vi "Error Code Processor.vi"() -> ()   [LabVIEW 2012]
uses:
  <vilib>/Utility/file.llb/Read From Spreadsheet File (string).vi
panel:
  in  "Typedef für Error Labels":path
  in  "Typedef für Error Codes":path
  in  "Btn_ReadErrorFromCsv":bool
  in  "ErrorTable":string[][](table) caption="Codetabelle"
  in  "Btn_SaveErrorToCtl":bool
  in  "Exit":bool
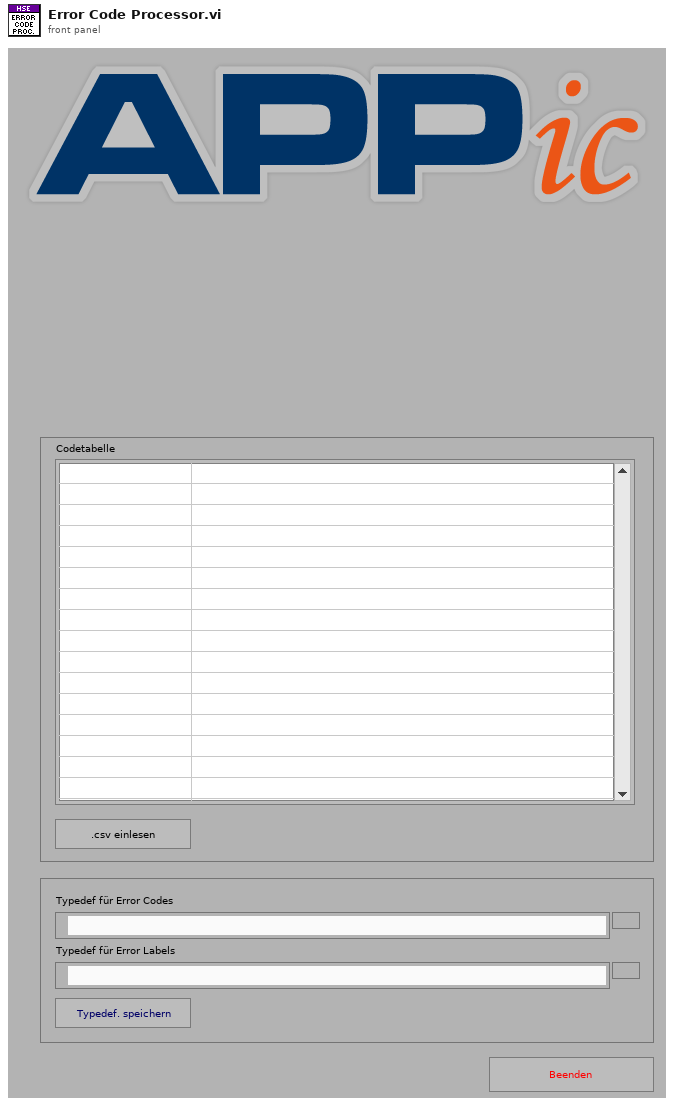
[diagram p1: front panel]
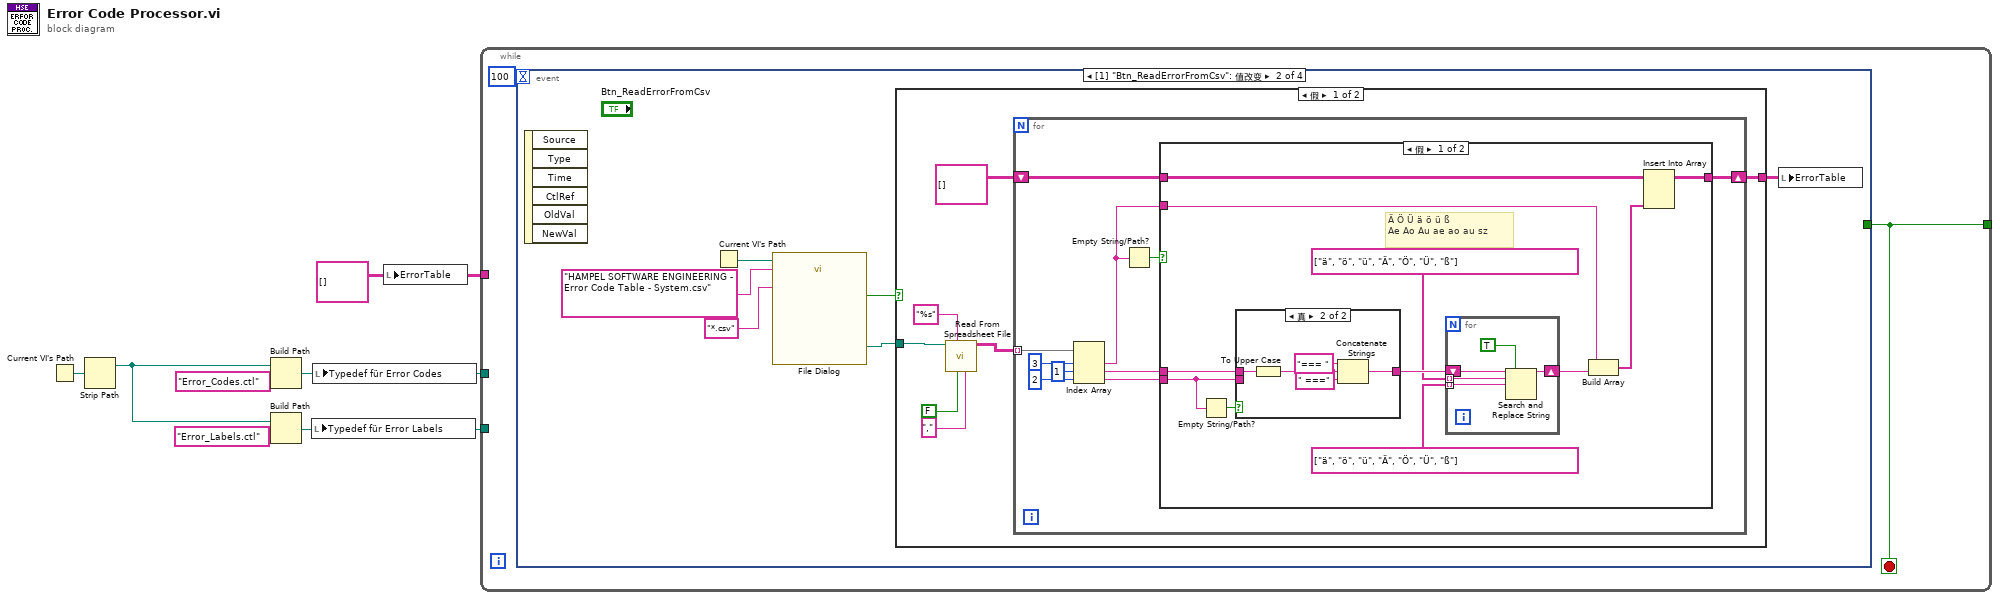
[diagram p0: block diagram]
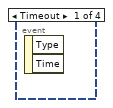
[diagram p2: hidden frame]
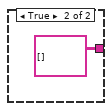
[diagram p5: hidden frame]
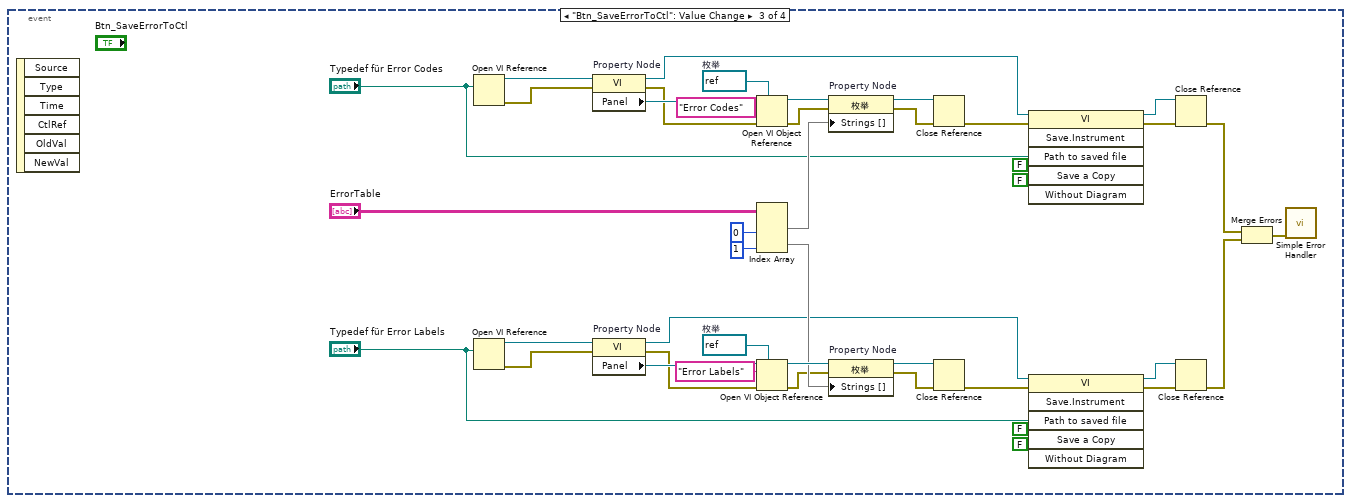
[diagram p6: hidden frame]
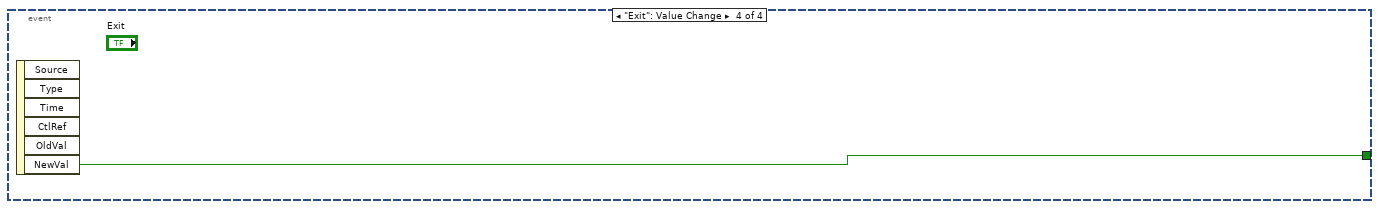
[diagram p7: hidden frame]
diagram:
  w7 = string[][] [] ("ErrorTable")
  n1 = Current VI's Path() -> (path=w6:path)
  n2 = Strip Path(path=w6) -> (stripped path=w1:path)  [unwired: 1 out]
  n3 = Build Path(base path=w1, name or relative path="Error_Codes.ctl") -> (appended path=w5:path)
  n4 = Build Path(base path=w1, name or relative path="Error_Labels.ctl") -> (appended path=w4:path)
  n5 = local write "Typedef für Error Labels"(w4) -> ()
  n6 = local write "Typedef für Error Codes"(w5) -> ()
  n7 = local write "ErrorTable"(w7) -> ()
  n8 = while {
    tunnel: [w9] -> _
    tunnel: w7 -> [_]
    tunnel: w5 -> [_]
    tunnel: w4 -> [_]
    stop <- w9 stop-if-true
    n9 = event shown="[1] \"Btn_ReadErrorFromCsv\": 值改变" {
      selector: _ -> [_ _ _ _]
      dyn-events: _ -> [_ _ _ _]
      timeout: 100 -> [_ _ _ _]
      tunnel: [_ _ _ w99] -> w9
      event Timeout {
        n10 = event-data() -> ()  [unwired: 3 out]
      }
      event "Btn_ReadErrorFromCsv": Value Change {
        n11 = event-data() -> ()  [unwired: 7 out]
        n12 = Current VI's Path() -> (path=w12:path)
        n13 = call "File Dialog"("start path"=w12, "default name"="HAMPEL SOFTWARE ENGINEERING - Error Code Table - System.csv", "pattern (all files)"="*.csv") -> ("selected path"=w14:path, "cancelled"=w13:bool)  [unwired: 9 in, 2 out]
        n14 = case shown="假" w13 {
          tunnel: [w17 string[][] []] -> w15
          tunnel: w14 -> [w16 _]
          frame False {
            n15 = call-poly <vilib>:"Read From Spreadsheet File.vi"("delimiter (\\t)"="," ("delimiter (\\t)"), "transpose (no:F)"=FALSE, "format (%s)"="%s", "file path (dialog if empty)"=w16) -> ("all rows"=w19:string[][])  [unwired: 3 in, 4 out]
            n16 = for {
              tunnel: w19 -> [w32] mode=indexing
              shift-right: [w27] -> w17
              shift-left: string[][] [] -> [w29]
              n17 = Index Array(array=w32, index #1=3 ("index"), index #2=1 ("index"), index #3=2 ("index")) -> (element #1=w25:string, element #2=w24:string, element #3=w23:string)
              n18 = Empty String/Path?(string/path=w25) -> (empty?=w28:bool)
              n19 = case shown="假" w28 {
                tunnel: w29 -> [w43 w55]
                tunnel: w25 -> [w37 _]
                tunnel: [w42 w55] -> w27
                tunnel: w24 -> [w38 _]
                tunnel: w23 -> [w39 _]
                frame False {
                  # "Ä Ö Ü ä ö ü ß\nAe Ao Au ae ao au sz"
                  n20 = Empty String/Path?(string/path=w39) -> (empty?=w40:bool)
                  n21 = case shown="真" w40 {
                    tunnel: w39 -> [w49 _]
                    tunnel: [w49 w53] -> w36
                    tunnel: w38 -> [_ w54]
                    frame False {
                    }
                    frame True {
                      n22 = To Upper Case(1:w54) -> (0:w50:string)
                      n23 = Concatenate Strings("=== " ("string"), w50, " ===" ("string")) -> (w53:string)
                    }
                  }
                  n24 = for {
                    tunnel: string[] ["ä", "ö", "ü", "Ä", "Ö", "Ü", "ß"] -> [w46] mode=indexing
                    shift-right: [w47] -> w35
                    shift-left: w36 -> [w48]
                    tunnel: string[] ["ä", "ö", "ü", "Ä", "Ö", "Ü", "ß"] -> [w45] mode=indexing
                    n25 = Search and Replace String(replace all?=TRUE ("replace all? (F)"), input string=w48, search string=w45, replace string=w46) -> (result string=w47:string)  [unwired: 4 in, 3 out]
                  }
                  n26 = Build Array(w37, w35) -> (w41:string[])
                  n27 = Insert Into Array(array=w43, new element=w41) -> (w42:string[][])  [unwired: 2 in]
                }
                frame True {
                }
              }
            }
          }
          frame True {
          }
        }
        n28 = local write "ErrorTable"(w15) -> ()
      }
      event "Btn_SaveErrorToCtl": Value Change {
        w91 = refnum<vi> refnum  # 枚举
        w94 = refnum<vi> refnum  # 枚举
        n29 = event-data() -> ()  [unwired: 7 out]
        n30 = Open VI Reference(vi path="Typedef für Error Codes") -> (vi reference=w88:refnum<vi>, error out=w87:errorcluster)  [unwired: 5 in]
        n31 = Open VI Reference(vi path="Typedef für Error Labels") -> (vi reference=w97:refnum<vi>, error out=w98:errorcluster)  [unwired: 5 in]
        n32 = property on="Property Node" class="VI"(reference=w88, error in=w87) -> (reference out=w69:refnum<vi>, error out=w82:errorcluster, "Panel"=w89:refnum<vi>)
        n33 = property on="Property Node" class="VI"(reference=w97, error in=w98) -> (reference out=w61:refnum<vi>, error out=w80:errorcluster, "Panel"=w96:refnum<vi>)
        n34 = Open VI Object Reference(7:w91, 8:w82, 10:"Error Codes" ("name/order"), 11:w89) -> (0:w81:errorcluster, 3:w92:refnum<vi>)
        n35 = Index Array(array="ErrorTable", index (col) #1=0 ("disabled index (col)"), index (col) #2=1 ("index (col)")) -> (element #1=w84:string[], element #2=w83:string[])  [unwired: 2 in]
        n36 = Open VI Object Reference(7:w94, 8:w80, 10:"Error Labels" ("name/order"), 11:w96) -> (0:w79:errorcluster, 3:w93:refnum<vi>)
        n37 = property on="Property Node" class="枚举"(reference=w92, error in=w81, "Strings []"=w84) -> (reference out=w72:refnum<vi>, error out=w78:errorcluster)
        n38 = property on="Property Node" class="枚举"(reference=w93, error in=w79, "Strings []"=w83) -> (reference out=w76:refnum<vi>, error out=w75:errorcluster)
        n39 = Close Reference(reference=w72, error in (no error)=w78) -> (error out=w71:errorcluster)
        n40 = Close Reference(reference=w76, error in (no error)=w75) -> (error out=w65:errorcluster)
        n41 = invoke class="VI" method="Save.Instrument"(reference=w69, error in=w71, "Path to saved file"="Typedef für Error Codes", "Save a Copy"=FALSE, "Without Diagram"=FALSE) -> (reference out=w68:refnum<vi>, error out=w70:errorcluster)  [unwired: 1 in, 4 out]
        n42 = invoke class="VI" method="Save.Instrument"(reference=w61, error in=w65, "Path to saved file"="Typedef für Error Labels", "Save a Copy"=FALSE, "Without Diagram"=FALSE) -> (reference out=w60:refnum<vi>, error out=w64:errorcluster)  [unwired: 1 in, 4 out]
        n43 = Close Reference(reference=w68, error in (no error)=w70) -> (error out=w77:errorcluster)
        n44 = Close Reference(reference=w60, error in (no error)=w64) -> (error out=w74:errorcluster)
        n45 = Merge Errors(w77, w74) -> (w73:errorcluster)
        n46 = call <vilib>:"Simple Error Handler.vi"("error in (no error)"=w73) -> ()  [unwired: 4 in, 5 out]
      }
      event "Exit": Value Change {
        n47 = event-data() -> ("NewVal"=w99:bool)  [unwired: 6 out]
      }
    }
  }
